vi "6509 Pnuematic Outputs_2.vi"(1 "device name":tag="Dev1", 2 "error in (no error)":errorcluster, 3 "Enable Output":bool, 4 "Enum":T1(ring)) -> (0 "error out":errorcluster)   [LabVIEW 2014]
panel:
  out "data 2":bool[](array[boolean])
  in  "data":bool[](array[boolean])
  # "Pos 4"
  # "pos 5"
  # "Pos 10"
  # "Pos 11"
  # "Pos 12"
  # "Pos 13"
  # "Pos 14"
  # "Pos 15"
  # "Pos 7"
  # "Pos 0"
  # "Pos 1"
  # "Pos 2"
  # "Pos 3"
  # "Pos 6"
  # "Pos 8"
  # "Pos 9"
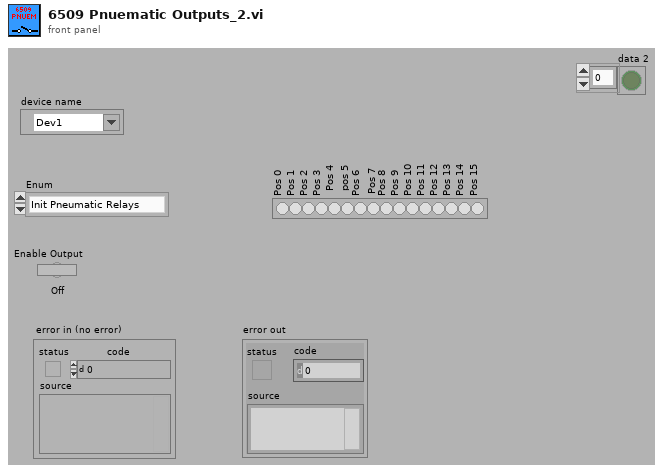
[diagram p1: front panel]
types:
  T1 = enum16{"Init Pneumatic Relays", "Pneumatic_Drive_0", "Pneumatic_Drive_1", "Pneumatic_Drive_2", "Pneumatic_Drive_3", "Pneumatic_Drive_4", "Pneumatic_Drive_5", "Pneumatic_Drive_6", "Pneumatic_Drive_7", "Pneumatic_Drive_8", "Pneumatic_Drive_9", "Pneumatic_Drive_10", "Pneumatic_Drive_11", "Pneumatic_Drive_12", "Pneumatic_Drive_13", "Pneumatic_Drive_14", "Pneumatic_Drive_15"}
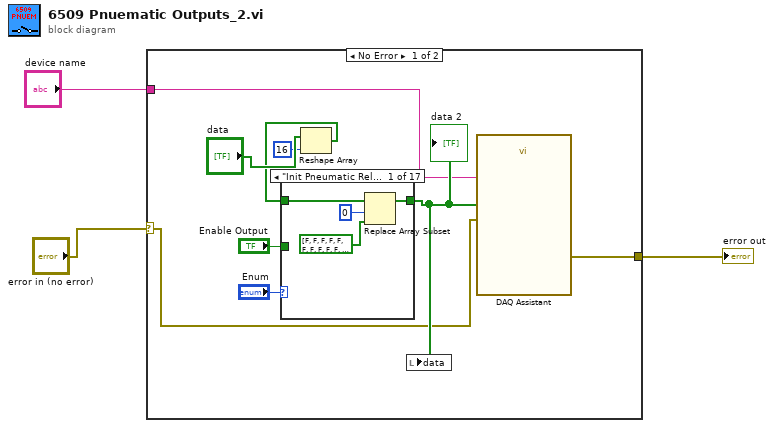
[diagram p0: block diagram]
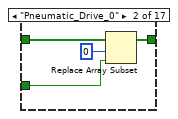
[diagram p2: hidden frame]
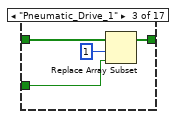
[diagram p3: hidden frame]
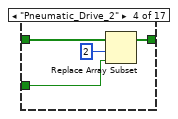
[diagram p4: hidden frame]
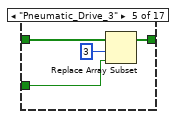
[diagram p5: hidden frame]
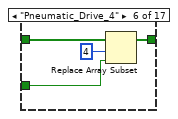
[diagram p6: hidden frame]
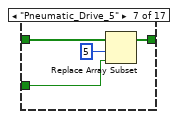
[diagram p7: hidden frame]
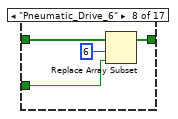
[diagram p8: hidden frame]
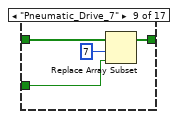
[diagram p9: hidden frame]
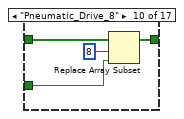
[diagram p10: hidden frame]
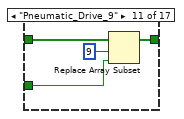
[diagram p11: hidden frame]
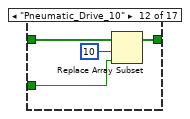
[diagram p12: hidden frame]
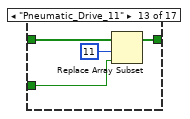
[diagram p13: hidden frame]
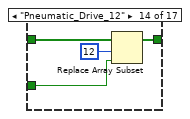
[diagram p14: hidden frame]
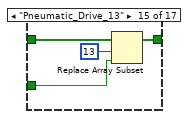
[diagram p15: hidden frame]
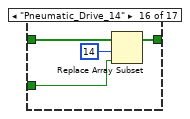
[diagram p16: hidden frame]
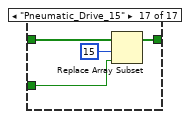
[diagram p17: hidden frame]
diagram:
  n1 = case shown="No Error" "error in (no error)" {
    selector: "error in (no error)" -> [w5 w81]
    tunnel: [w11 w81] -> w3
    tunnel: "device name" -> [w4 _]
    frame No Error {
      n2 = Reshape Array("data", 16 ("dimension size")) -> (w7:bool[])
      n3 = case shown="\"Init Pneumatic Relays\", Default" "Enum" {
        tunnel: "Enable Output" -> [_ w20 w22 w26 w30 w34 w38 w42 w46 w50 w54 w58 w62 w66 w70 w74 w78]
        tunnel: w7 -> [w16 w19 w23 w27 w31 w35 w39 w43 w47 w51 w55 w59 w63 w67 w71 w75 w79]
        tunnel: [w14 w17 w21 w25 w29 w33 w37 w41 w45 w49 w53 w57 w61 w65 w69 w73 w77] -> w6
        frame "Init Pneumatic Relays", Default {
          n4 = Replace Array Subset(array=w16, new element=bool[] [FALSE, FALSE, FALSE, FALSE, FALSE, FALSE, FALSE, FALSE, FALSE, FALSE, FALSE, FALSE, FALSE, FALSE, FALSE, FALSE] ("data 2"), index=0) -> (w14:bool[])
        }
        frame "Pneumatic_Drive_0" {
          n5 = Replace Array Subset(array=w19, new element=w20, index=0) -> (w17:bool[])
        }
        frame "Pneumatic_Drive_1" {
          n6 = Replace Array Subset(array=w23, new element=w22, index=1) -> (w21:bool[])
        }
        frame "Pneumatic_Drive_2" {
          n7 = Replace Array Subset(array=w27, new element=w26, index=2) -> (w25:bool[])
        }
        frame "Pneumatic_Drive_3" {
          n8 = Replace Array Subset(array=w31, new element=w30, index=3) -> (w29:bool[])
        }
        frame "Pneumatic_Drive_4" {
          n9 = Replace Array Subset(array=w35, new element=w34, index=4) -> (w33:bool[])
        }
        frame "Pneumatic_Drive_5" {
          n10 = Replace Array Subset(array=w39, new element=w38, index=5) -> (w37:bool[])
        }
        frame "Pneumatic_Drive_6" {
          n11 = Replace Array Subset(array=w43, new element=w42, index=6) -> (w41:bool[])
        }
        frame "Pneumatic_Drive_7" {
          n12 = Replace Array Subset(array=w47, new element=w46, index=7) -> (w45:bool[])
        }
        frame "Pneumatic_Drive_8" {
          n13 = Replace Array Subset(array=w51, new element=w50, index=8) -> (w49:bool[])
        }
        frame "Pneumatic_Drive_9" {
          n14 = Replace Array Subset(array=w55, new element=w54, index=9) -> (w53:bool[])
        }
        frame "Pneumatic_Drive_10" {
          n15 = Replace Array Subset(array=w59, new element=w58, index=10) -> (w57:bool[])
        }
        frame "Pneumatic_Drive_11" {
          n16 = Replace Array Subset(array=w63, new element=w62, index=11) -> (w61:bool[])
        }
        frame "Pneumatic_Drive_12" {
          n17 = Replace Array Subset(array=w67, new element=w66, index=12) -> (w65:bool[])
        }
        frame "Pneumatic_Drive_13" {
          n18 = Replace Array Subset(array=w71, new element=w70, index=13) -> (w69:bool[])
        }
        frame "Pneumatic_Drive_14" {
          n19 = Replace Array Subset(array=w75, new element=w74, index=14) -> (w73:bool[])
        }
        frame "Pneumatic_Drive_15" {
          n20 = Replace Array Subset(array=w79, new element=w78, index=15) -> (w77:bool[])
        }
      }
      "data 2" <- w6
      n21 = local write "data"(w6) -> ()
      n22 = call "DAQ Assistant"("data"=w6, "error in"=w5, "device name"=w4) -> ("error out"=w11:errorcluster)  [unwired: 15 in, 1 out]
    }
    frame Error {
    }
  }
  "error out" <- w3
